vi "Save As Sif.vi"(8 "error in (no error)":errorcluster, 11 "path":string) -> (0 "error out":errorcluster, 2 "function return":u32, 3 "path out":string)   [LabVIEW 2014, in "atmcd32d.lvlib"]
doc: "unsigned int WINAPI SaveAsSif(char * path);"
uses:
  atmcd32d.lvlib
  atmcd32d.dll
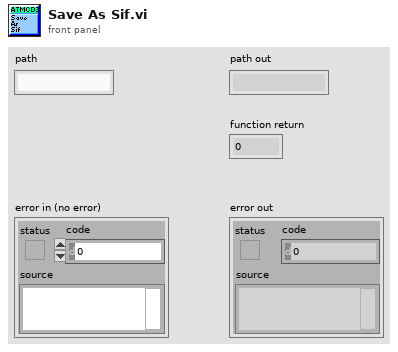
[diagram p1: front panel]
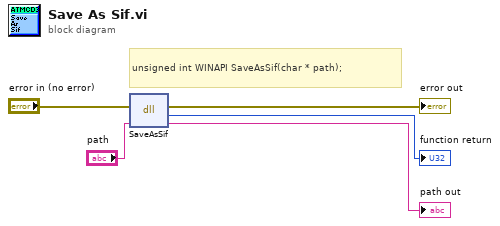
[diagram p0: block diagram]
diagram:
  # "unsigned int WINAPI SaveAsSif(char * path);"
  n1 = dll-call lib="C:/Users/Bakir/Documents/Lambda2-Testing/lib/Andorlib/atmcd32d.*" fn="SaveAsSif"(error in="error in (no error)", "path"="path") -> (error out=→"error out":errorcluster, →"function return":u32, "path"=→"path out":string)  [unwired: 2 in, 1 out]
